vi "test_WFRamp.vi"() -> ()   [LabVIEW 2013]
uses:
  random/impl/RandomArray_D.vi
panel:
  out "Result Waveform 3":waveform(dbl)(graph)={"t0"=timestamp(0 s since 1904-01-01), "dt"=0.001, "Y"=array[5001 elements]}
  in  "Ramp 3":dbl=2.5
  out "Result Waveform 2":waveform(dbl)(graph)={"t0"=timestamp(0 s since 1904-01-01), "dt"=0.001, "Y"=array[5001 elements]}
  in  "Ramp 2":dbl=0.1
  out "Result Waveform 1":waveform(dbl)(graph)={"t0"=timestamp(0 s since 1904-01-01), "dt"=0.001, "Y"=array[5001 elements]}
  in  "Ramp 1":dbl
  out "Start Waveform":waveform(dbl)(graph)={"t0"=timestamp(0 s since 1904-01-01), "dt"=0.001, "Y"=array[5001 elements]}
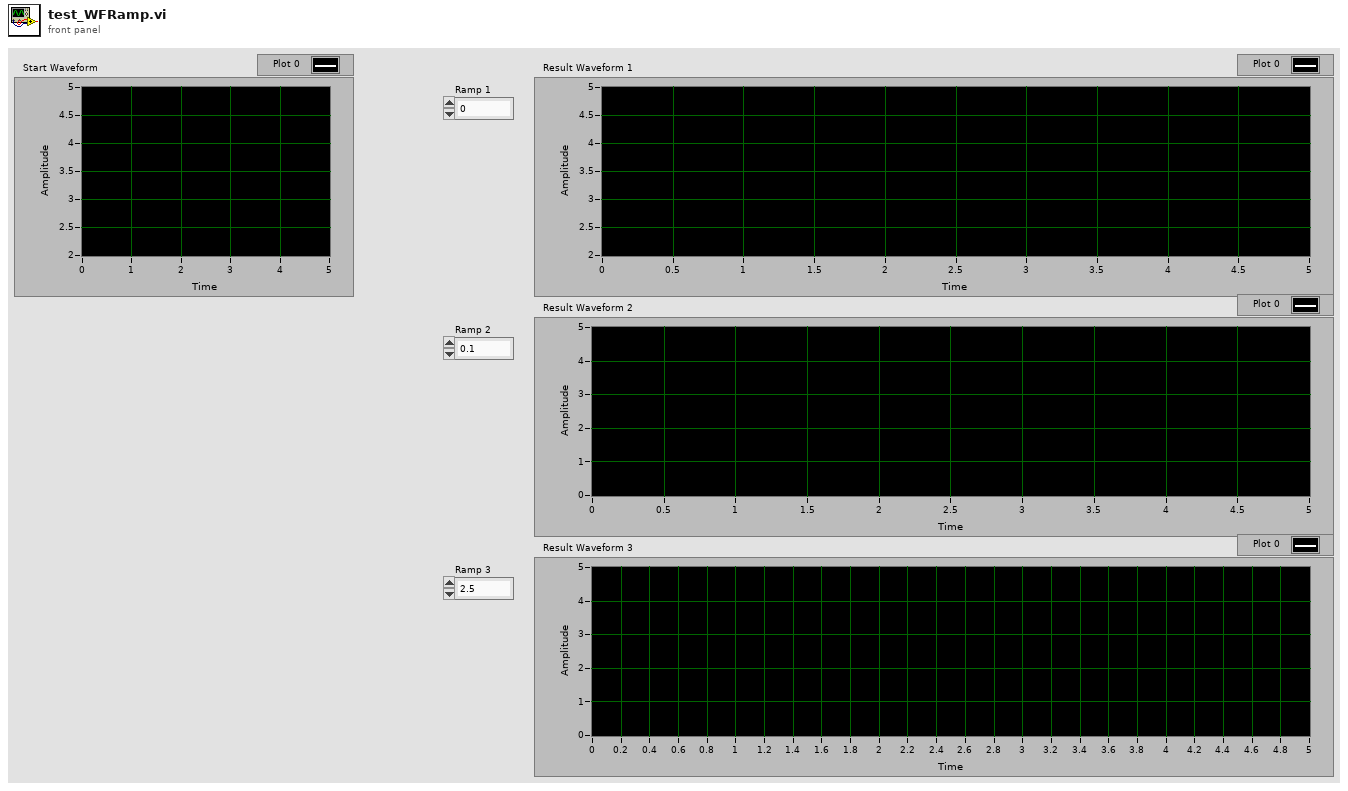
[diagram p1: front panel]
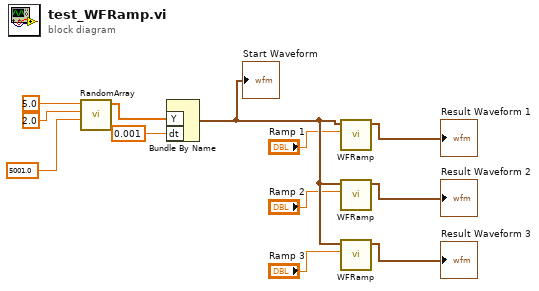
[diagram p0: block diagram]
diagram:
  n1 = call-poly "RandomArray.vi"("N"=5001.0, "Min"=2.0, "Max 2"=5.0 ("Max")) -> ("Array"=w8:dbl[])  [unwired: 8 in]
  n2 = Bundle By Name("Y"=w8, "dt"=0.001) -> (w7:waveform(dbl))  [unwired: 1 in]
  "Start Waveform" <- w7
  n3 = call "WFRamp.vi"("Ramp Length (s)"="Ramp 1", "Waveform In"=w7) -> ("Waveform Out"=→"Result Waveform 1":waveform(dbl))  [unwired: 8 in, 1 out]
  n4 = call "WFRamp.vi"("Ramp Length (s)"="Ramp 2", "Waveform In"=w7) -> ("Waveform Out"=→"Result Waveform 2":waveform(dbl))  [unwired: 8 in, 1 out]
  n5 = call "WFRamp.vi"("Ramp Length (s)"="Ramp 3", "Waveform In"=w7) -> ("Waveform Out"=→"Result Waveform 3":waveform(dbl))  [unwired: 8 in, 1 out]
